vi "Setup Path Group.vi"(0 "Path Group in":refnum<class "Path Group.lvclass">, 11 "error in":errorcluster) -> (4 "Path Group out":refnum<class "Path Group.lvclass">, 6 "Path Callbacks Reference":refnum<vi>[](array[refnum]), 15 "error out":errorcluster)   [LabVIEW 2023, in "RFCalAndFixtureCharact.Common.lvlib"]
uses:
  RFCalAndFixtureCharact.Common.lvlib
  Base Classes/Path Group/Path Group.lvclass
  Base Classes/Path/Path.lvclass
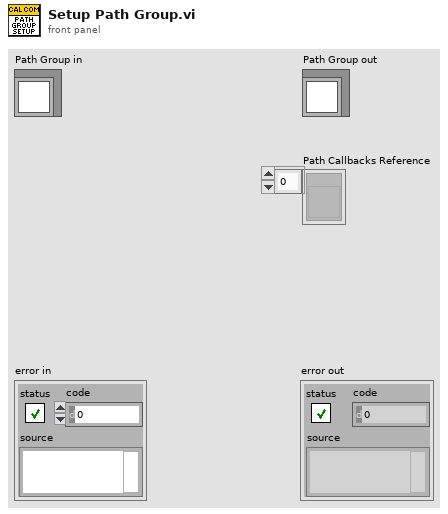
[diagram p1: front panel]
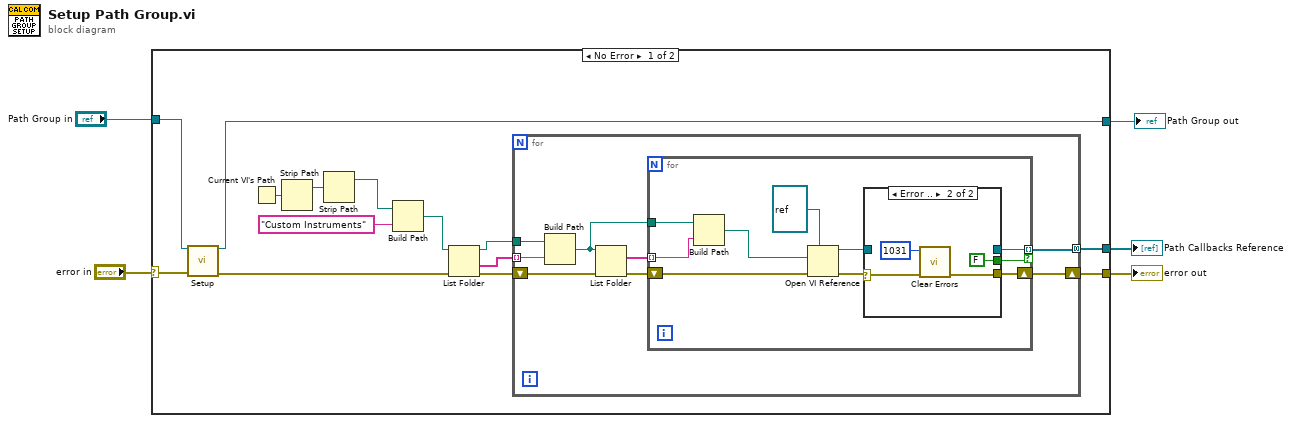
[diagram p0: block diagram]
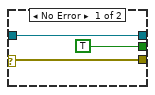
[diagram p2: hidden frame]
diagram:
  n1 = case shown="No Error" "error in" {
    selector: "error in" -> [w14 w46]
    tunnel: [w16 w46] -> w4
    tunnel: "Path Group in" -> [w13 w45]
    tunnel: [w12 w45] -> w2
    tunnel: [w6 _] -> w1
    frame No Error {
      n2 = call-dynamic "Setup.vi"("Path Group in"=w13, "error in"=w14) -> ("Path Group out"=w12:refnum<class "Path Group.lvclass">, "error out"=w11:errorcluster)  [unwired: 12 in]
      n3 = Current VI's Path() -> (path=w18:path)
      n4 = Strip Path(path=w18) -> (stripped path=w19:path)  [unwired: 1 out]
      n5 = Strip Path(path=w19) -> (stripped path=w15:path)  [unwired: 1 out]
      n6 = Build Path(base path=w15, name or relative path="Custom Instruments") -> (appended path=w9:path)
      n7 = List Folder(path=w9, error in=w11) -> (path out=w7:path, folder names=w8:string[], error out=w10:errorcluster)  [unwired: 2 in, 1 out]
      n8 = for {
        shift-right: [w27] -> w16
        shift-left: w10 -> [w24]
        tunnel: w8 -> [w23] mode=indexing
        tunnel: w7 -> [w22]
        tunnel: [w20] -> w6 mode=concatenating
        n9 = Build Path(base path=w22, name or relative path=w23) -> (appended path=w21:path)
        n10 = List Folder(path=w21, error in=w24) -> (filenames=w26:string[], error out=w25:errorcluster)  [unwired: 2 in, 2 out]
        n11 = for {
          tunnel: w26 -> [w36] mode=indexing
          tunnel: w21 -> [w37]
          shift-right: [w31] -> w27
          shift-left: w25 -> [w35]
          tunnel: [w29] -> w20 mode=indexing if=w28
          n12 = Build Path(base path=w37, name or relative path=w36) -> (appended path=w34:path)
          n13 = Open VI Reference(type specifier VI Refnum (for type only)=refnum<vi> refnum, vi path=w34, error in (no error)=w35) -> (vi reference=w30:refnum<vi>, error out=w32:errorcluster)  [unwired: 3 in]
          n14 = case shown="Error .." w32 {
            selector: w32 -> [w40 w44]
            tunnel: [w40 w43] -> w31
            tunnel: w30 -> [w39 _]
            tunnel: [w39 _] -> w29
            tunnel: [TRUE FALSE] -> w28
            frame No Error {
            }
            frame Error {
              n15 = call <vilib>:"Clear Errors.vi"("error in (no error)"=w44, "specific error code to clear (0: all)"=1031) -> ("error out"=w43:errorcluster)  [unwired: 4 in, 1 out]
            }
          }
        }
      }
    }
    frame Error {
    }
  }
  "error out" <- w4
  "Path Group out" <- w2
  "Path Callbacks Reference" <- w1
